vi "wa32 PeekNamedPipe.vi"(8 "error in":errorcluster, 10 "bytes to read (0)":i32, 11 "handle":i32) -> (0 "error out":errorcluster, 1 "read bytes":u32, 2 "read data":u8[](array[numeric]), 3 "handle out":i32, 4 "string data":string, 5 "available bytes":u32)   [LabVIEW 2013]
doc: "WinAPI PeekNamedPipe() wrapper. Non-destructive read of pipe data and returns also total available read bytes count in the pipe."
uses:
  <vilib>/Utility/error.llb/Error Cluster From Error Code.vi
  <vilib>/ErrorRing/Error Ring.xnode
  kernel32.dll
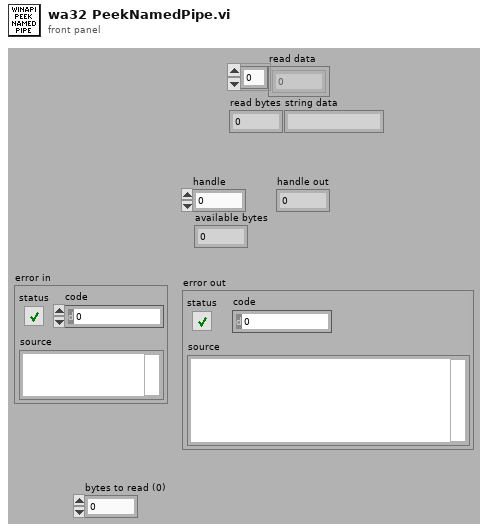
[diagram p1: front panel]
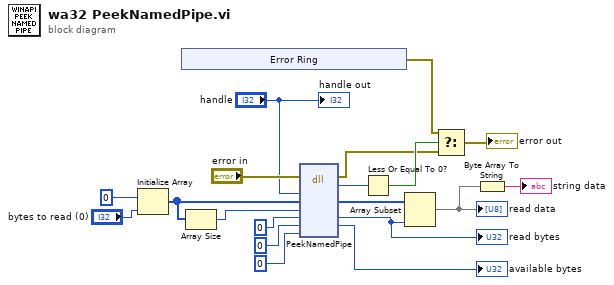
[diagram p0: block diagram]
diagram:
  n1 = Initialize Array(u8 0, "bytes to read (0)") -> (w5:u8[])
  n2 = xnode "Error Ring"() -> ("error out"=w14:errorcluster)
  n3 = Array Size(array=w5) -> (size(s)=w6:i32)
  n4 = dll-call lib="kernel32.dll" fn="PeekNamedPipe"(error in="error in", "handle"="handle", "data"=w5, "toRead"=w6, "read"=u32 0 ("available"), "available"=u32 0 ("data"), "leftMsg"=u32 0 ("overlapped")) -> (error out=w16:errorcluster, "errout"=w18:i32, "data"=w4:u8[], "read"=w3:u32, "available"=→"available bytes":u32)  [unwired: 5 in, 1 out]
  "read bytes" <- w3
  n5 = Less Or Equal To 0?(x=w18) -> (x <= 0?=w17:bool)
  n6 = Array Subset(array=w4, length=w3) -> (w2:u8[])  [unwired: 1 in]
  "read data" <- w2
  n7 = Select(t=w14, s=w17, f=w16) -> (s? t:f=→"error out":errorcluster)
  n8 = Byte Array To String(unsigned byte array=w2) -> (string=→"string data":string)
  "handle out" <- "handle"
